vi "Fast Set Multiple Dependent Node Refs FuncGlobal2.vi"(5 "Action":enum16{"Open or Add", "Close Ref"}(ring), 8 "error in (no error)":errorcluster, 9 "Dependent Node Refs":T1[](array[typedef]) format="%.0x", 10 "Base Property Name":string, 11 "Item Ref in":T1 format="%.0x") -> (0 "error out":errorcluster, 3 "Item Ref out":T1=18446744073709551615 format="%.0x")   [LabVIEW 2011]
uses:
  <vilib>/NI Veristand/Custom Device API/Custom Device Item Ref.ctl
  <vilib>/NI Veristand/Custom Device API/Get Item Property (Variant).vi
  <vilib>/NI Veristand/Custom Device API/Set Item Property (Variant).vi
  <vilib>/NI Veristand/Custom Device API/Custom Device API.lvlib
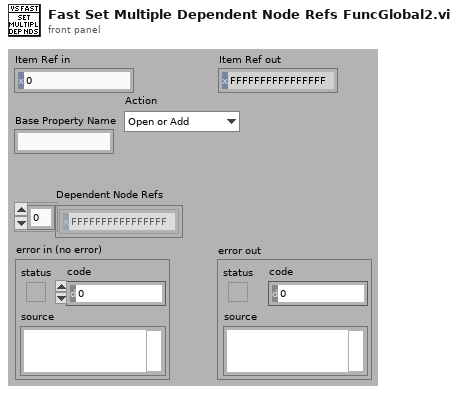
[diagram p1: front panel]
types:
  T1 = typedef "Custom Device API.lvlib/Custom Device Item Ref.ctl" = u64
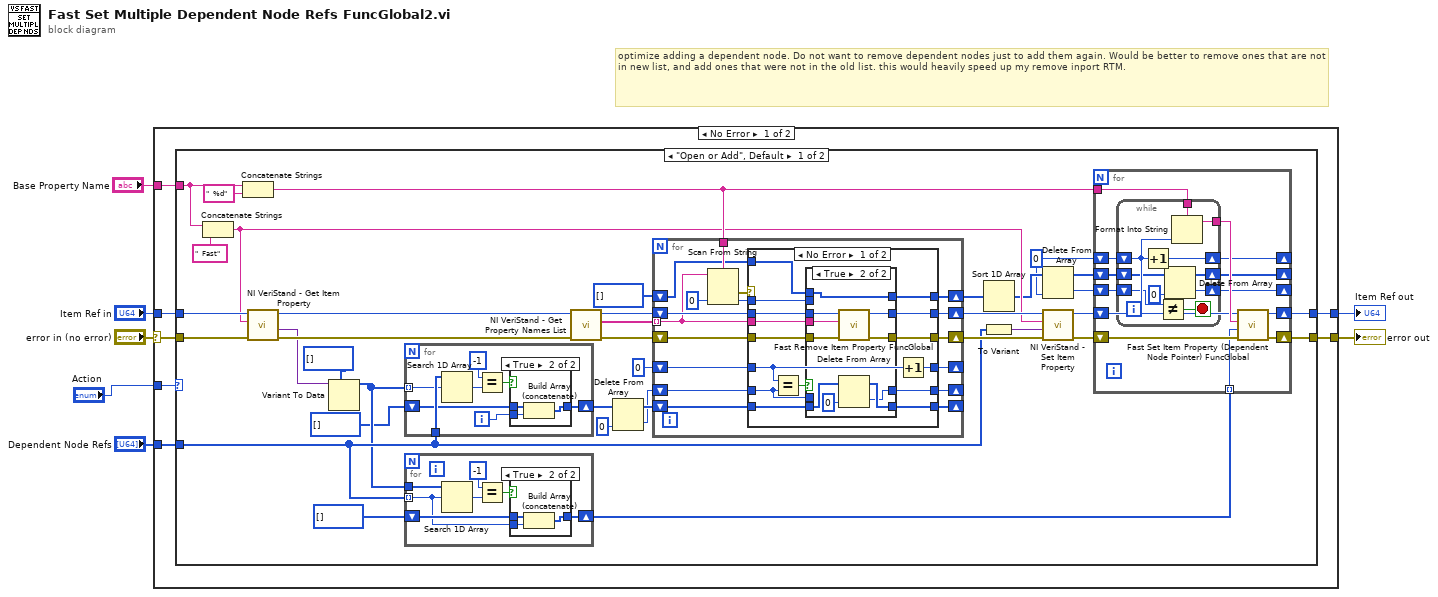
[diagram p0: block diagram]
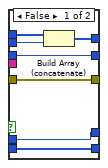
[diagram p4: hidden frame]
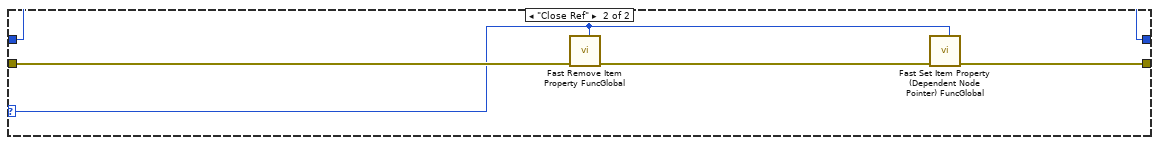
[diagram p6: hidden frame]
diagram:
  # "optimize adding a dependent node. Do not want to remove dependent nodes just to add them again. Would be better to remove ones that are not in new list, and add ones that were not in the old list. this would heavily speed up my remove inport RTM."
  n1 = case shown="No Error" "error in (no error)" {
    selector: "error in (no error)" -> [w9 w158]
    tunnel: "Item Ref in" -> [w14 w159]
    tunnel: "Dependent Node Refs" -> [w13 _]
    tunnel: [w12 w159] -> w5
    tunnel: [w11 w158] -> w4
    tunnel: "Base Property Name" -> [w10 _]
    tunnel: "Action" -> [w8 _]
    frame No Error {
      n2 = case shown="\"Open or Add\", Default" w8 {
        selector: w8 -> [_ w156]
        tunnel: w14 -> [w35 w153]
        tunnel: w13 -> [w30 _]
        tunnel: [w48 w153] -> w12
        tunnel: [w47 w154] -> w11
        tunnel: w10 -> [w38 _]
        tunnel: w9 -> [w37 w157]
        frame "Open or Add", Default {
          w15 = 0 ("default value 1")
          n3 = Concatenate Strings(w38, "  Fast" ("string")) -> (w33:string)
          n4 = Concatenate Strings(w38, "  %d" ("string")) -> (w44:string)
          n5 = call-poly <vilib>:"NI VeriStand - Get Item Property.vi"("error in (no error)"=w37, "Property Name"=w33, "Item Ref in"=w35) -> ("error out"=w36:errorcluster, "Value"=w31:variant, "Item Ref out"=w34:T1)  [unwired: 5 in, 1 out]
          n6 = Variant To Data(type=T1[] [] ("Dependent Node Refs"), Variant=w31) -> (data=w28:T1[])  [unwired: 1 in, 1 out]
          n7 = for {
            tunnel: w28 -> [w66] mode=indexing
            tunnel: w30 -> [w70]
            shift-right: [w65] -> w25
            shift-left: i32[] [] -> [w64]
            i -> [w63]
            n8 = Search 1D Array(1D array=w70, element=w66) -> (index of element=w69:i32)  [unwired: 1 in]
            n9 = Equal?(x=-1, y=w69) -> (x = y?=w67:bool)
            n10 = case shown="True" w67 {
              tunnel: w63 -> [_ w74]
              tunnel: [w71 w73] -> w65
              tunnel: w64 -> [w71 w72]
              frame False {
              }
              frame True {
                n11 = Build Array (concatenate)(w72, w74) -> (w73:i32[])
              }
            }
          }
          n12 = for {
            tunnel: w30 -> [w52] mode=indexing
            shift-right: [w55] -> w27
            shift-left: T1[] [] -> [w54]
            tunnel: w28 -> [w53]
            n13 = Search 1D Array(1D array=w53, element=w52) -> (index of element=w58:i32)  [unwired: 1 in]
            n14 = Equal?(x=-1, y=w58) -> (x = y?=w56:bool)
            n15 = case shown="True" w56 {
              tunnel: w52 -> [_ w62]
              tunnel: [w59 w61] -> w55
              tunnel: w54 -> [w59 w60]
              frame False {
              }
              frame True {
                n16 = Build Array (concatenate)(w60, w62) -> (w61:T1[])
              }
            }
          }
          n17 = call <vilib>:"NI VeriStand - Get Property Names List.vi"("error in (no error)"=w36, "Item Ref in"=w34) -> ("error out"=w50:errorcluster, "Property Names"=w49:string[], "Item Ref out"=w51:T1)  [unwired: 7 in]
          n18 = Delete From Array(array=w25, index=0) -> (deleted portion=w23:i32, array with subset deleted=w24:i32[])  [unwired: 1 in]
          n19 = for {
            shift-right: [w110] -> w43
            shift-left: w50 -> [w112]
            tunnel: w49 -> [w111] mode=indexing
            shift-right: [w109] -> w41
            shift-left: w51 -> [w114]
            tunnel: w44 -> [w108]
            shift-right: [w105] -> _
            shift-left: 0 ("default value 1") -> [w106]
            shift-right: [w102] -> _
            shift-left: w24 -> [w104]
            shift-right: [w101] -> _
            shift-left: w23 -> [w103]
            shift-right: [w99] -> w20
            shift-left: i32[] [] -> [w98]
            n20 = Scan From String(format string=w108, input string=w111, default 1=0 ("default value 1")) -> (error out=w113:errorcluster, output 1=w100:i32)  [unwired: 2 in, 2 out]
            n21 = case shown="No Error" w113 {
              tunnel: w114 -> [w127 w151]
              tunnel: w112 -> [w129 w152]
              tunnel: w111 -> [w128 _]
              tunnel: [w125 w152] -> w110
              tunnel: [w126 w151] -> w109
              tunnel: w106 -> [w123 w150]
              tunnel: [w124 w150] -> w105
              tunnel: w104 -> [w121 w149]
              tunnel: w103 -> [w118 w148]
              tunnel: [w120 w149] -> w102
              tunnel: [w119 w148] -> w101
              tunnel: w100 -> [w117 _]
              tunnel: [w116 w147] -> w99
              tunnel: w98 -> [w115 w147]
              frame No Error {
                n22 = Equal?(x=w123, y=w118) -> (x = y?=w122:bool)
                n23 = case shown="True" w122 {
                  tunnel: w129 -> [w136 w146]
                  tunnel: w128 -> [_ w145]
                  tunnel: w127 -> [w135 w144]
                  tunnel: [w135 w143] -> w126
                  tunnel: [w136 w142] -> w125
                  tunnel: w121 -> [w134 w141]
                  tunnel: [w134 w140] -> w120
                  tunnel: [w133 w139] -> w119
                  tunnel: w118 -> [w133 _]
                  tunnel: w117 -> [w132 _]
                  tunnel: [w131 w138] -> w116
                  tunnel: w115 -> [w130 w138]
                  frame False {
                    n24 = Build Array (concatenate)(w130, w132) -> (w131:i32[])
                  }
                  frame True {
                    n25 = call "Fast Remove Item Property FuncGlobal.vi"("error in (no error)"=w146, "Property Name"=w145, "Item Ref in"=w144) -> ("error out"=w142:errorcluster, "Item Ref out"=w143:T1)  [unwired: 6 in, 1 out]
                    n26 = Delete From Array(array=w141, index=0) -> (deleted portion=w139:i32, array with subset deleted=w140:i32[])  [unwired: 1 in]
                  }
                }
                n27 = Increment(x=w123) -> (x+1=w124:i32)
              }
              frame Error {
              }
            }
          }
          n28 = Sort 1D Array(array=w20) -> (sorted array=w19:i32[])
          n29 = To Variant(anything=w30) -> (Variant=w39:variant)
          n30 = Delete From Array(array=w19, index=w15) -> (deleted portion=w17:i32, array with subset deleted=w18:i32[])  [unwired: 1 in]
          n31 = call-poly <vilib>:"NI VeriStand - Set Item Property.vi"("error in (no error)"=w43, "Value"=w39, "Property Name"=w33, "Item Ref in"=w41) -> ("error out"=w42:errorcluster, "Item Ref out"=w40:T1)  [unwired: 5 in, 1 out]
          n32 = for {
            shift-right: [w81] -> w47
            shift-left: w42 -> [w86]
            tunnel: w44 -> [w87]
            shift-right: [w82] -> w48
            shift-left: w40 -> [w83]
            tunnel: w27 -> [w85] mode=indexing
            shift-right: [w75] -> _
            shift-left: w15 -> [w80]
            shift-right: [w76] -> _
            shift-left: w18 -> [w79]
            shift-right: [w77] -> _
            shift-left: w17 -> [w78]
            n33 = while {
              tunnel: w87 -> [w97]
              tunnel: [w96] -> w84
              shift-right: [w90] -> w76
              shift-left: w79 -> [w91]
              shift-right: [w89] -> w77
              shift-left: w78 -> [w92]
              shift-right: [w94] -> w75
              shift-left: w80 -> [w93]
              stop <- w95 stop-if-true
              n34 = Increment(x=w93) -> (x+1=w94:i32)
              n35 = Not Equal?(x=w92, y=w93) -> (x != y?=w95:bool)
              n36 = Delete From Array(array=w91, index=0) -> (deleted portion=w89:i32, array with subset deleted=w90:i32[])  [unwired: 1 in]
              n37 = Format Into String(format string=w97, w93) -> (resulting string=w96:string)  [unwired: 2 in, 1 out]
            }
            n38 = call "Fast Set Item Property (Dependent Node Pointer) FuncGlobal.vi"("error in (no error)"=w86, "Dependent Node Ref"=w85, "Property Name"=w84, "Item Ref in"=w83) -> ("error out"=w81:errorcluster, "Item Ref out"=w82:T1)  [unwired: 5 in, 1 out]
          }
        }
        frame "Close Ref" {
          n39 = call "Fast Remove Item Property FuncGlobal.vi"("Action"=w156, "error in (no error)"=w157) -> ("error out"=w155:errorcluster)  [unwired: 7 in, 2 out]
          n40 = call "Fast Set Item Property (Dependent Node Pointer) FuncGlobal.vi"("Action"=w156, "error in (no error)"=w155) -> ("error out"=w154:errorcluster)  [unwired: 7 in, 2 out]
        }
      }
    }
    frame Error {
    }
  }
  "Item Ref out" <- w5
  "error out" <- w4
